vi "Configure Math Function Source.vi"(5 "Math Function Index (1: Math Function 1)":i32(ring)=1 items=["Math Function 1"=1, "Math Function 2"=2, "Math Function 3"=3, "Math Function 4"=4], 6 "Signal Source 2 (4: None)":i32(ring)=4 items=["Channel 1", "Channel 2", "Channel 3", "Channel 4", "None", "Waveform Memory 1", "Waveform Memory 2"], 7 "Signal Source 1 (0: Channel 1)":i32(ring) items=["Channel 1", "Channel 2", "Channel 3", "Channel 4", "GOFT", "Bus 1", "Bus 2", "Function 1", "Function 2", "Function 3", "Math 1", "Math 2", "Math 3", "Waveform Memory 1", "Waveform Memory 2"], 8 "error in (no error)":errorcluster, 9 "GOFT Source 2 (1: Channel 2)":i32(ring)=1 items=["Channel 1", "Channel 2", "Channel 3", "Channel 4"], 10 "GOFT Source 1 (0: Channel 1)":i32(ring) items=["Channel 1", "Channel 2", "Channel 3", "Channel 4"], 11 "VISA resource name":refnum<visa-resource-name>) -> (0 "error out":errorcluster, 3 "VISA resource name out":refnum<visa-resource-name>)   [LabVIEW 2015, in "Agilent 2000 3000 X-Series.lvlib"]
doc: "Configures the math function source."
uses:
  Agilent 2000 3000 X-Series.lvlib
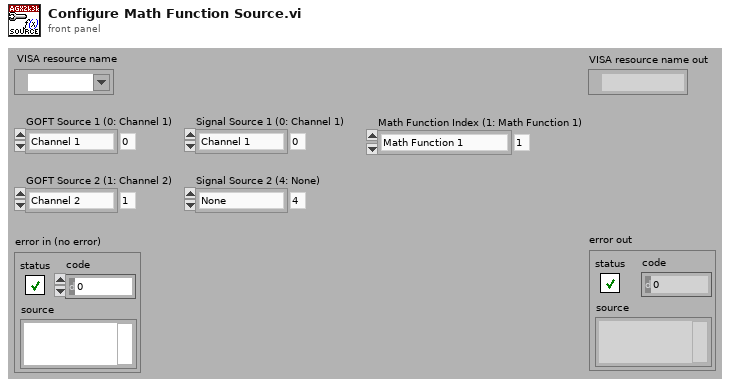
[diagram p1: front panel]
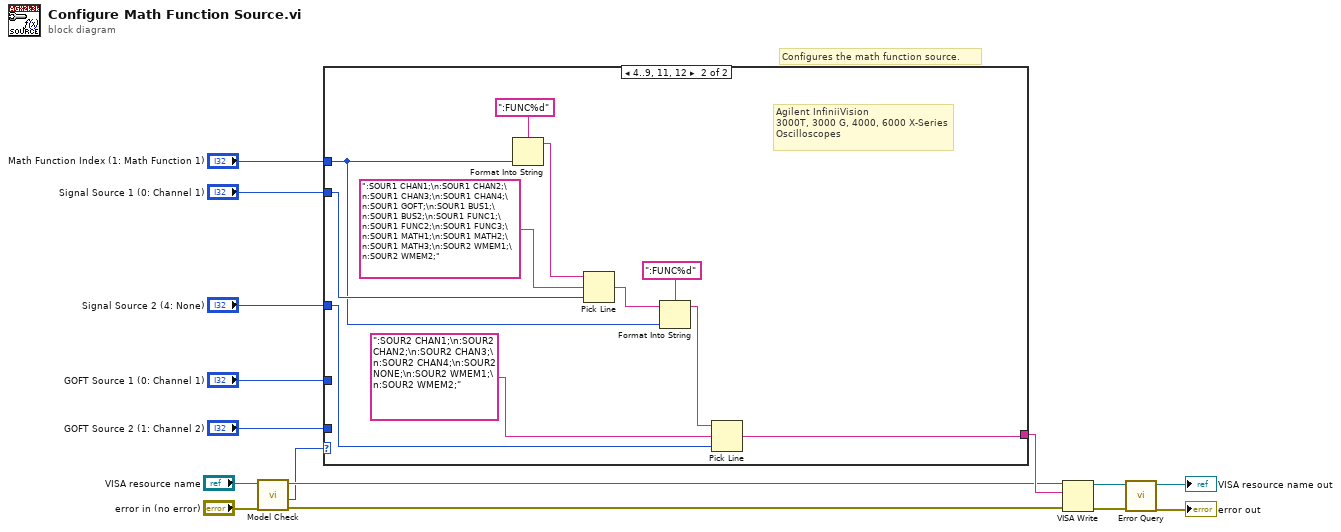
[diagram p0: block diagram]
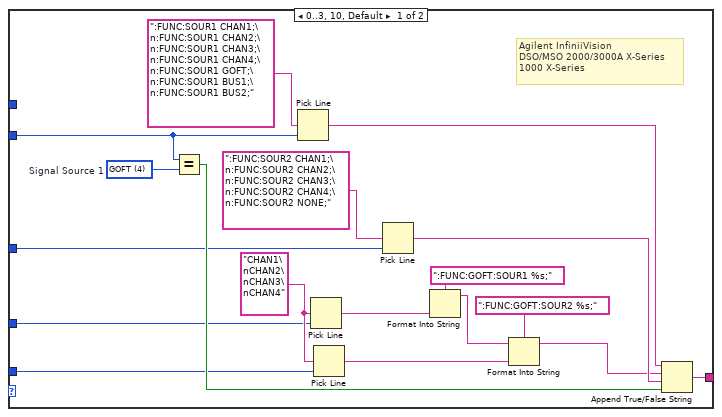
[diagram p2: hidden frame]
diagram:
  # "Configures the math function source."
  n1 = call "Model Check.vi"("error in (no error)"="error in (no error)", "VISA resource name"="VISA resource name") -> ("error out"=w2:errorcluster, "Model"=w1:i32, "VISA resource name out"=w3:refnum<visa-resource-name>)  [unwired: 7 out]
  n2 = case shown="4..9, 11, 12" w1 {
    tunnel: "Signal Source 1 (0: Channel 1)" -> [w21 w40]
    tunnel: "Signal Source 2 (4: None)" -> [w20 w34]
    tunnel: "GOFT Source 1 (0: Channel 1)" -> [w19 _]
    tunnel: "GOFT Source 2 (1: Channel 2)" -> [w18 _]
    tunnel: [w17 w36] -> w6
    tunnel: "Math Function Index (1: Math Function 1)" -> [_ w35]
    frame 0..3, 10, Default {
      w16 = 4 items=["Channel 1", "Channel 2", "Channel 3", "Channel 4", "GOFT"]  # Signal Source 1
      w33 = "CHAN1\nCHAN2\nCHAN3\nCHAN4"
      # "Agilent InfiniiVision\nDSO/MSO 2000/3000A X-Series\n1000 X-Series"
      n3 = Equal?(x=w21, y=w16) -> (x = y?=w27:bool)
      n4 = Pick Line(multi-line string=":FUNC:SOUR1 CHAN1;\n:FUNC:SOUR1 CHAN2;\n:FUNC:SOUR1 CHAN3;\n:FUNC:SOUR1 CHAN4;\n:FUNC:SOUR1 GOFT;\n:FUNC:SOUR1 BUS1;\n:FUNC:SOUR1 BUS2;", line index=w21) -> (output string=w29:string)  [unwired: 1 out]
      n5 = Pick Line(multi-line string=w33, line index=w19) -> (output string=w31:string)  [unwired: 1 out]
      n6 = Pick Line(multi-line string=w33, line index=w18) -> (output string=w32:string)  [unwired: 1 out]
      n7 = Pick Line(multi-line string=":FUNC:SOUR2 CHAN1;\n:FUNC:SOUR2 CHAN2;\n:FUNC:SOUR2 CHAN3;\n:FUNC:SOUR2 CHAN4;\n:FUNC:SOUR2 NONE;", line index=w20) -> (output string=w30:string)  [unwired: 1 out]
      n8 = Format Into String(format string=":FUNC:GOFT:SOUR1 %s;", w31) -> (resulting string=w25:string)  [unwired: 2 in, 1 out]
      n9 = Format Into String(format string=":FUNC:GOFT:SOUR2 %s;", initial string=w25, w32) -> (resulting string=w28:string)  [unwired: 1 in, 1 out]
      n10 = Append True/False String(1:w27, 2:w30, 3:w28, 4:w29) -> (0:w17:string)
    }
    frame 4..9, 11, 12 {
      # "Agilent InfiniiVision\n3000T, 3000 G, 4000, 6000 X-Series\nOscilloscopes"
      n11 = Format Into String(format string=":FUNC%d", w35) -> (resulting string=w41:string)  [unwired: 2 in, 1 out]
      n12 = Pick Line(string ("")=w41, multi-line string=":SOUR1 CHAN1;\n:SOUR1 CHAN2;\n:SOUR1 CHAN3;\n:SOUR1 CHAN4;\n:SOUR1 GOFT;\n:SOUR1 BUS1;\n:SOUR1 BUS2;\n:SOUR1 FUNC1;\n:SOUR1 FUNC2;\n:SOUR1 FUNC3;\n:SOUR1 MATH1;\n:SOUR1 MATH2;\n:SOUR1 MATH3;\n:SOUR2 WMEM1;\n:SOUR2 WMEM2;", line index=w40) -> (output string=w38:string)
      n13 = Format Into String(format string=":FUNC%d", initial string=w38, w35) -> (resulting string=w37:string)  [unwired: 1 in, 1 out]
      n14 = Pick Line(string ("")=w37, multi-line string=":SOUR2 CHAN1;\n:SOUR2 CHAN2;\n:SOUR2 CHAN3;\n:SOUR2 CHAN4;\n:SOUR2 NONE;\n:SOUR2 WMEM1;\n:SOUR2 WMEM2;", line index=w34) -> (output string=w36:string)
    }
  }
  n15 = VISA Write(VISA resource name=w3, write buffer=w6, error in (no error)=w2) -> (VISA resource name out=w15:refnum<visa-resource-name>, error out=w14:errorcluster)  [unwired: 1 out]
  n16 = call "Error Query.vi"("error in (no error)"=w14, "VISA resource name"=w15) -> ("error out"=→"error out":errorcluster, "VISA resource name out"=→"VISA resource name out":refnum<visa-resource-name>)  [unwired: 8 out]
